vi "Initialize.vi"(8 "error in (no error)":errorcluster, 11 "UI in":refnum<class "UI.lvclass">) -> (0 "error out":errorcluster, 3 "UI out":refnum<class "UI.lvclass">, 4 "Event Registration Refnum":T1)   [LabVIEW 2020, in "AR Example.lvlib" / "UI.lvclass"]
uses:
  UI.lvclass
  UI.lvclass/UI.ctl
  Stop Event.ctl
  Events.ctl
  Event Registration.ctl
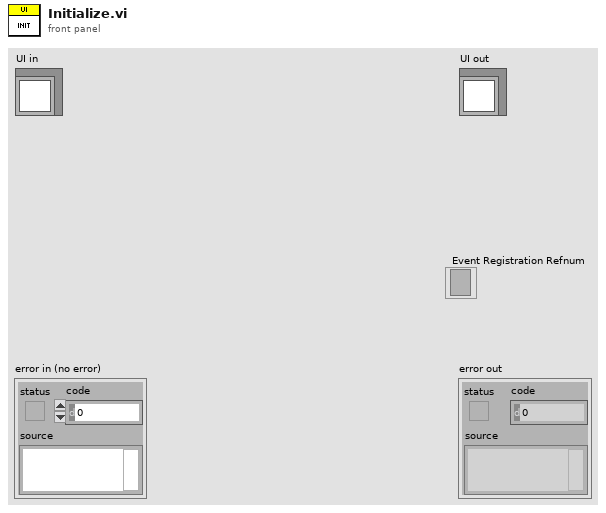
[diagram p1: front panel]
types:
  T1 = typedef "AR Example.lvlib/UI.lvclass/Event Registration.ctl" = refnum<event-registration>
  T2 = typedef "AR Example.lvlib/UI.lvclass/Events.ctl" = cluster{"Stop":refnum<user-event>}
  T3 = typedef "AR Example.lvlib/UI.lvclass/Stop Event.ctl" = cluster{"Data":bool}
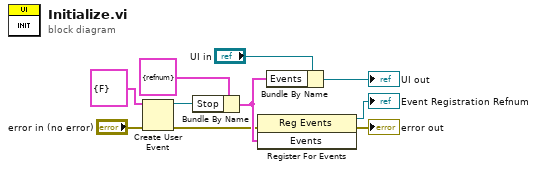
[diagram p0: block diagram]
diagram:
  n1 = Create User Event(user event datatype=T3 {"Data"=FALSE} ("Stop"), error in="error in (no error)") -> (user event=w8:refnum<user-event>, error out=w2:errorcluster)
  n2 = Bundle By Name(cluster=T2 {"Stop"=refnum} ("Events"), "Stop"=w8) -> (w4:T2)
  n3 = register-events(error in=w2, w4) -> (reference out=→"Event Registration Refnum":refnum<event-registration>, error out=→"error out":errorcluster)  [unwired: 1 in]
  n4 = Bundle By Name(cluster="UI in", "Events"=w4) -> (→"UI out":refnum<class "UI.lvclass">)
